vi "Vaportubes.vi"() -> ()   [LabVIEW 2018]
uses:
  <resource>/objmgr/daqmx.rc
panel:
  in  "index 2":i32=2
  in  "index":i32=1
  in  "Temperature Task":refnum<k21>="TC1"
  in  "Refresh Time (ms)":u32=50
  out "appended array":waveform(dbl)[](graph)
  in  "stop":bool
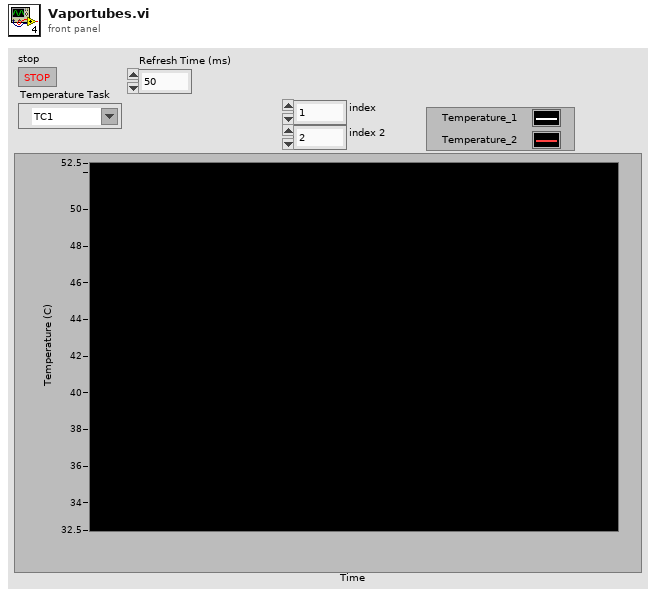
[diagram p1: front panel]
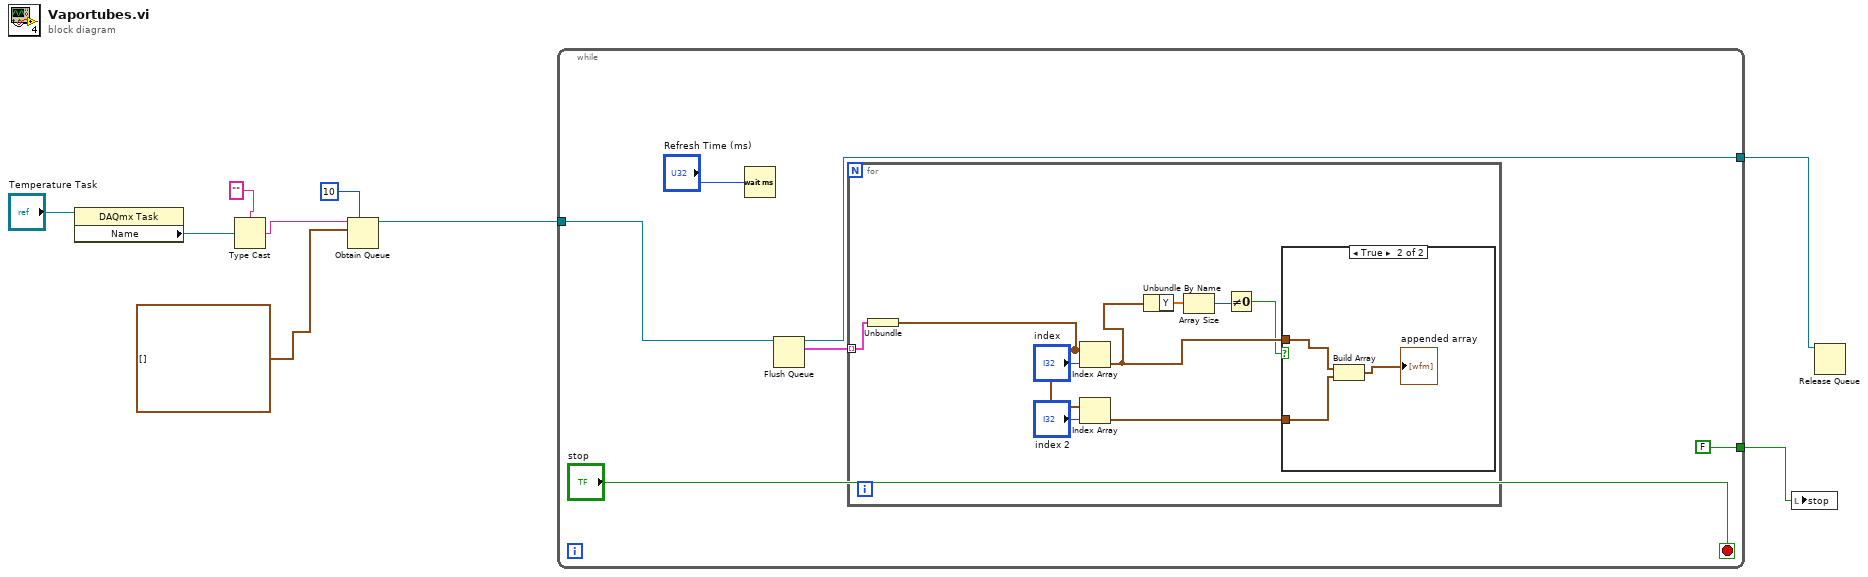
[diagram p0: block diagram]
diagram:
  n1 = property class="DAQmx Task"(reference="Temperature Task") -> ("Name"=w8:refnum<k21>)  [unwired: 1 in, 2 out]
  n2 = Type Cast(type="", x=w8) -> (*(type *) &x=w6:string)
  n3 = Obtain Queue(max queue size (-1, unlimited)=10, name (unnamed)=w6, element data type=waveform(dbl)[] [] ("data")) -> (queue out=w3:refnum<queue>)  [unwired: 2 in, 2 out]
  n4 = while {
    tunnel: [FALSE] -> w9
    tunnel: w3 -> [w13]
    tunnel: [w12] -> w1
    stop <- "stop" stop-if-true
    n5 = Wait (ms)(milliseconds to wait="Refresh Time (ms)") -> ()  [unwired: 1 out]
    n6 = Flush Queue(queue=w13) -> (queue out=w12:refnum<queue>, remaining elements=w10:cluster{"data":waveform(dbl)[]}[])  [unwired: 1 in, 1 out]
    n7 = for {
      tunnel: w10 -> [w17] mode=indexing
      n8 = Unbundle(w17) -> ("data"=w16:waveform(dbl)[])
      n9 = Index Array(array=w16, index="index") -> (element=w23:waveform(dbl))
      n10 = Index Array(array=w16, index="index 2") -> (element=w24:waveform(dbl))
      n11 = Unbundle By Name(w23) -> ("Y"=w22:dbl[])
      n12 = Array Size(array=w22) -> (size(s)=w21:i32)
      n13 = Not Equal To 0?(x=w21) -> (x != 0?=w20:bool)
      n14 = case shown="True" w20 {
        tunnel: w24 -> [_ w27]
        tunnel: w23 -> [_ w25]
        frame False {
        }
        frame True {
          n15 = Build Array(w25, w27) -> (→"appended array":waveform(dbl)[])
        }
      }
    }
  }
  n16 = local write "stop"(w9) -> ()
  n17 = Release Queue(queue=w1) -> ()  [unwired: 2 in, 3 out]
